vi "Do Main Action.vi"(8 "error in (no error)":errorcluster, 10 "AbstractData":refnum<class "AbstractData.lvclass">, 11 "AbstractExtractor in":refnum<class "AbstractExtractor.lvclass">) -> (0 "error out":errorcluster, 3 "AbstractExtractor out":refnum<class "AbstractExtractor.lvclass">)   [LabVIEW 2014, in "AbstractExtractor.lvclass"]
uses:
  AbstractExtractor.lvclass
  Model/Data/AbstractData/AbstractData.lvclass
  Interfaces/Pipelined Actor/Pipelined Actor.lvclass
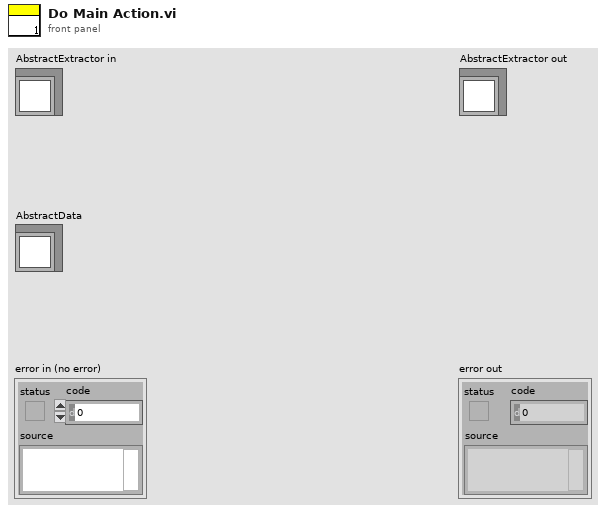
[diagram p1: front panel]
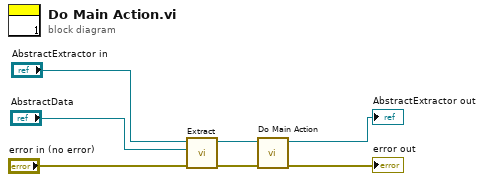
[diagram p0: block diagram]
diagram:
  n1 = call-dynamic "Extract.vi"("error in (no error)"="error in (no error)", "AbstractData in"="AbstractData", "AbstractExtractor in"="AbstractExtractor in") -> ("error out"=w1:errorcluster, "AbstractExtractor out"=w2:refnum<class "AbstractExtractor.lvclass">)  [unwired: 7 in]
  n2 = call-parent "Do Main Action.vi"("error in (no error)"=w1, "Pipelined Actor in"=w2) -> ("error out"=→"error out":errorcluster, "Pipelined Actor out"=→"AbstractExtractor out":refnum<class "AbstractExtractor.lvclass">)  [unwired: 8 in]
